vi "Get Ctl Value.vi"(8 "error in (no error)":errorcluster, 11 "Numeric Field in":refnum<class "Numeric Field.lvclass">) -> (0 "error out":errorcluster, 2 "Value":string, 3 "Numeric Field out":refnum<class "Numeric Field.lvclass">)   [LabVIEW 2020, in "Numeric Field.lvclass"]
uses:
  Numeric Field.lvclass
  <vilib>/Utility/Data Type/NI_Data Type.lvlib
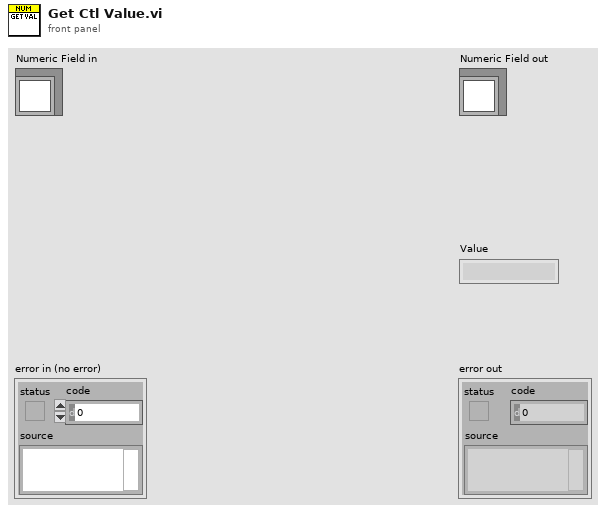
[diagram p1: front panel]
types:
  T1 = typedef "LVNumericRepresentation.ctl" = enum32{"Extended Precision", "Double Precision", "Single Precision", "Long", "Word", "Byte", "Unsigned Long", "Unsigned Word", "Unsigned Byte", "Complex Extended", "Complex Double", "Complex Single", "Quad", "Unsigned Quad", "Fixed-Point"}
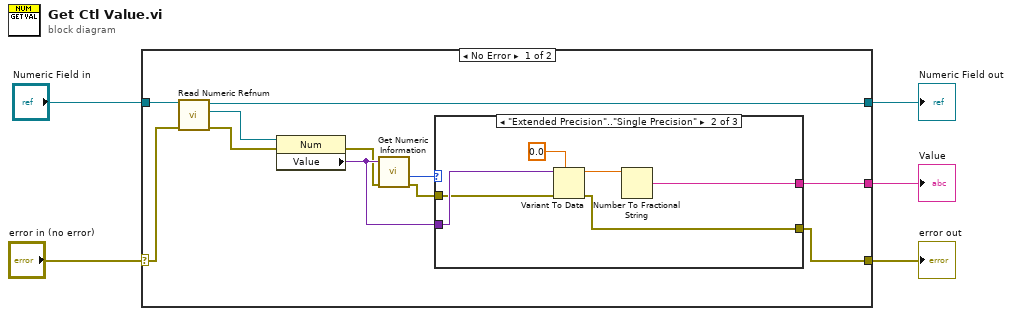
[diagram p0: block diagram]
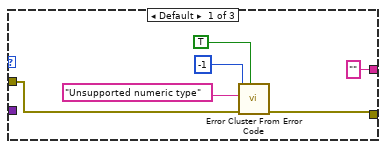
[diagram p2: hidden frame]
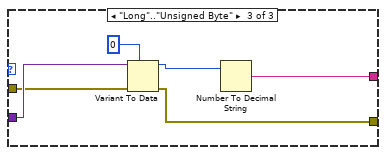
[diagram p3: hidden frame]
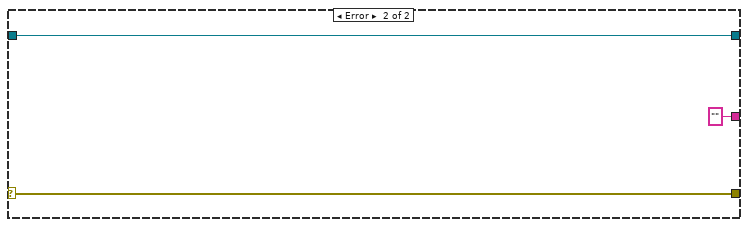
[diagram p4: hidden frame]
diagram:
  n1 = case shown="No Error" "error in (no error)" {
    selector: "error in (no error)" -> [w13 w37]
    tunnel: [w6 w37] -> w4
    tunnel: "Numeric Field in" -> [w16 w36]
    tunnel: [w15 w36] -> w2
    tunnel: [w8 ""] -> w1
    frame No Error {
      n2 = call "Read Numeric Refnum.vi"("error in (no error)"=w13, "Numeric Field in"=w16) -> ("error out"=w12:errorcluster, "Num Refnum"=w14:refnum<vi>, "Numeric Field out"=w15:refnum<class "Numeric Field.lvclass">)  [unwired: 7 in]
      n3 = property class="Num"(reference=w14, error in=w12) -> (error out=w10:errorcluster, "Value"=w11:variant)  [unwired: 1 out]
      n4 = call <vilib>:"Get Numeric Information.vi"("error in (no error)"=w10, "variant"=w11) -> ("error out"=w7:errorcluster, "representation"=w9:T1)  [unwired: 6 in, 2 out]
      n5 = case shown="\"Extended Precision\"..\"Single Precision\"" w9 {
        tunnel: w11 -> [_ w28 w34]
        tunnel: ["" w25 w29] -> w8
        tunnel: w7 -> [w20 w24 w32]
        tunnel: [w19 w23 w31] -> w6
        frame Default {
          n6 = call <vilib>:"Error Cluster From Error Code.vi"("show call chain? (False)"=TRUE, "error in (no error)"=w20, "error message (\"\")"="Unsupported numeric type" ("error message (\"\")"), "error code (0)"=-1) -> ("error out"=w19:errorcluster)  [unwired: 5 in]
        }
        frame "Extended Precision".."Single Precision" {
          n7 = Variant To Data(error in=w24, type=0.0, Variant=w28) -> (data=w26:dbl, error out=w23:errorcluster)
          n8 = Number To Fractional String(number=w26) -> (F-format string=w25:string)  [unwired: 3 in]
        }
        frame "Long".."Unsigned Byte" {
          n9 = Variant To Data(error in=w32, type=0, Variant=w34) -> (data=w30:i32, error out=w31:errorcluster)
          n10 = Number To Decimal String(number=w30) -> (decimal integer string=w29:string)  [unwired: 1 in]
        }
      }
    }
    frame Error {
    }
  }
  "error out" <- w4
  "Numeric Field out" <- w2
  "Value" <- w1
